vi "Load Package Arrays from File.vi"(3 "File name":string) -> (0 "Path Identifier Array":string[](array[string]), 1 "Package Name Array":string[](array[string]))   [LabVIEW 2019, in "Project.Dependencies Finder.lvlib"]
uses:
  Project.Dependencies Finder.lvlib
  5a637ef1-0df5-441d-8e21-cd64dd29224e.vi
  <vilib>/Utility/file.llb/Read Delimited Spreadsheet (string).vi
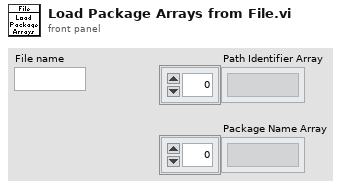
[diagram p1: front panel]
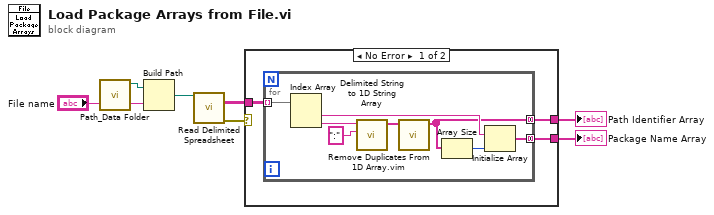
[diagram p0: block diagram]
diagram:
  n1 = call "Path_Data Folder.vi"() -> ("Data Folder Path"=w1:path)  [unwired: 11 in]
  n2 = Build Path(base path=w1, name or relative path="File name") -> (appended path=w3:path)
  n3 = call-poly <vilib>:"Read Delimited Spreadsheet.vi"("file path (dialog if empty)"=w3) -> ("all rows"=w5:string[][], "error out"=w4:errorcluster)  [unwired: 9 in, 4 out]
  n4 = case shown="No Error" w4 {
    tunnel: w5 -> [w10 _]
    tunnel: [w9 _] -> w6
    tunnel: [w8 _] -> w7
    frame No Error {
      n5 = for {
        tunnel: w10 -> [w18] mode=indexing
        tunnel: [w13] -> w8 mode=concatenating
        tunnel: [w11] -> w9 mode=concatenating
        n6 = Index Array(array=w18) -> (element #1=w14:string, element #2=w17:string)  [unwired: 2 in]
        n7 = call <vilib>:"Delimited String to 1D String Array.vi"("delimiter"=":", "delimited string"=w17) -> ("string array"=w12:string[])  [unwired: 9 in]
        n8 = call "Remove Duplicates From 1D Array.vim"("array"=w12) -> ("array with duplicates removed"=w11:string[])  [unwired: 10 in]
        n9 = Array Size(array=w11) -> (size(s)=w15:i32)
        n10 = Initialize Array(w14, w15) -> (w13:string[])
      }
    }
    frame Error {
    }
  }
  "Package Name Array" <- w7
  "Path Identifier Array" <- w6
